vi "Write_Multiple_ERD.vi"(0 "session in":refnum<k35>, 5 "Board":u8, 7 "dst":i64, 9 "Write ERD":T1 {"ERD" format="%x"}, 11 "error out":errorcluster) -> (4 "session out":refnum<k35>, 8 "Multiple Read":T3 {"ERD Number" format="%x"}, 15 "error IO":errorcluster)   [LabVIEW 2021]
uses:
  Controles/Multiple_Read_ERD.ctl
  Controles/Read_ERD.ctl
  Controles/Write_Multiple_ERD.ctl
  Controles/Write_ERD.ctl
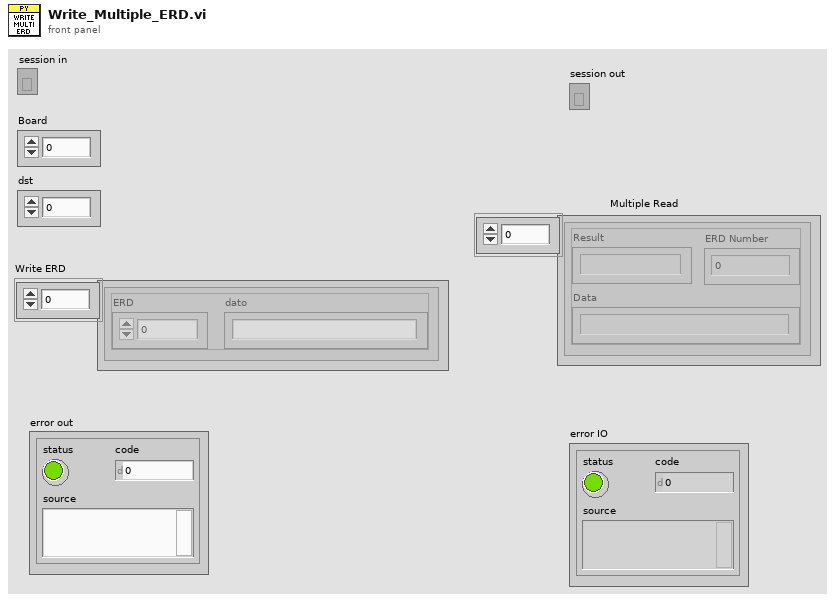
[diagram p1: front panel]
types:
  T1 = typedef "Write_Multiple_ERD.ctl" = T2[]
  T2 = typedef "Write_ERD.ctl" = cluster{"ERD":i64, "dato":string}
  T3 = typedef "Multiple_Read_ERD.ctl" = T4[]
  T4 = typedef "Read_ERD.ctl" = cluster{"Result":string, "ERD Number":i64, "Data":string}
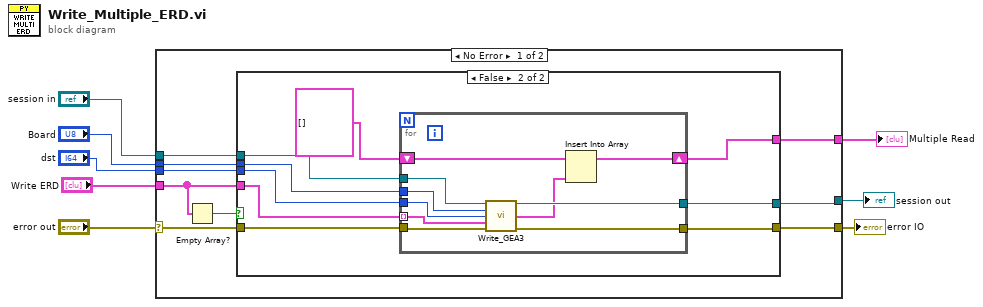
[diagram p0: block diagram]
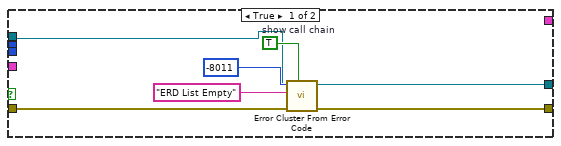
[diagram p2: hidden frame]
diagram:
  n1 = case shown="No Error" "error out" {
    selector: "error out" -> [w14 w43]
    tunnel: "Write ERD" -> [w12 _]
    tunnel: "session in" -> [w17 w44]
    tunnel: "Board" -> [w16 _]
    tunnel: "dst" -> [w15 _]
    tunnel: [w11 w43] -> w1
    tunnel: [w10 _] -> w4
    tunnel: [w9 w44] -> w3
    frame No Error {
      n2 = Empty Array?(array=w12) -> (empty?=w13:bool)
      n3 = case shown="False" w13 {
        tunnel: w12 -> [_ w32]
        tunnel: w17 -> [w19 w30]
        tunnel: w16 -> [_ w29]
        tunnel: w15 -> [_ w28]
        tunnel: w14 -> [w20 w27]
        tunnel: [w18 w25] -> w11
        tunnel: [_ w26] -> w10
        tunnel: [w19 w24] -> w9
        frame True {
          w23 = TRUE  # show call chain
          n4 = call <vilib>:"Error Cluster From Error Code.vi"("show call chain? (False)"=w23, "error in (no error)"=w20, "error message (\"\")"="ERD List Empty" ("error message (\"\")"), "error code (0)"=-8011) -> ("error out"=w18:errorcluster)  [unwired: 5 in]
        }
        frame False {
          n5 = for {
            tunnel: w29 -> [w38]
            tunnel: w28 -> [w37]
            tunnel: w30 -> [w36]
            tunnel: w32 -> [w39] mode=indexing
            shift-right: [w41] -> w26
            shift-left: T3 [] ("Multiple Read") -> [w42]
            tunnel: w27 -> [w40]
            tunnel: [w35] -> w25
            tunnel: [w34] -> w24
            n6 = call "Write_GEA3.vi"("session in"=w36, "board"=w38, "dst"=w37, "Write cluster"=w39, "error in (no error)"=w40) -> ("session out"=w34:refnum<k35>, "Write ERD"=w33:T4, "error out"=w35:errorcluster)  [unwired: 8 in]
            n7 = Insert Into Array(array=w42, new element=w33) -> (w41:T3)  [unwired: 1 in]
          }
        }
      }
    }
    frame Error {
    }
  }
  "Multiple Read" <- w4
  "error IO" <- w1
  "session out" <- w3
